vi "PickeringWriteConfig Asynchronous.vi"(8 "error in (no error)":errorcluster, 10 "Pickering Config":T1, 11 "Control Experiment in":refnum<class "Control Experiment.lvclass">) -> (0 "error out":errorcluster, 3 "Control Experiment out":refnum<class "Control Experiment.lvclass">)   [LabVIEW 2016, in "Control Experiment.lvclass"]
uses:
  Control Experiment.lvclass
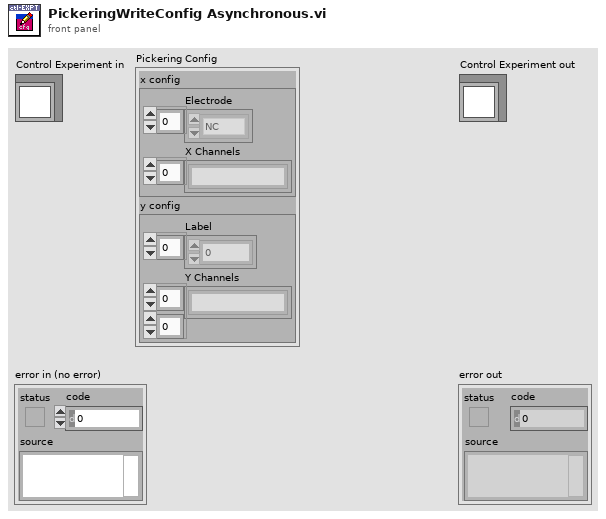
[diagram p1: front panel]
types:
  T1 = cluster{"x config":cluster{"Electrode":enum16{"NC", "26", "27", "28", "1", "2", "3", "4", "5", "6", "7", "8", "9", "10", "11", "12", "13", "14", "15", "16", "17", "18", "19", "20", "21", "22", "23", "24", "25"}[], "X Channels":string[]}, "y config":cluster{"Label":u16[], "Y Channels":string[][]}}
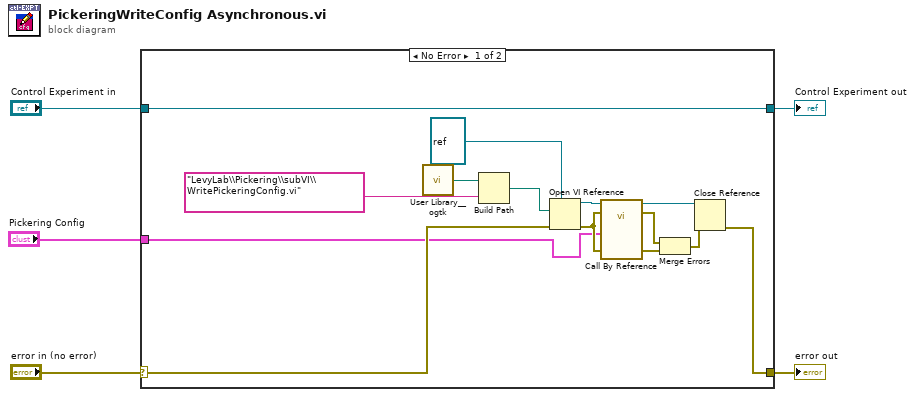
[diagram p0: block diagram]
diagram:
  n1 = case shown="No Error" "error in (no error)" {
    selector: "error in (no error)" -> [w9 w21]
    tunnel: [w8 w21] -> w4
    tunnel: [w19 w20] -> w2
    tunnel: "Control Experiment in" -> [w19 w20]
    tunnel: "Pickering Config" -> [w6 _]
    frame No Error {
      n2 = call <userlib>:"User Library__ogtk.vi"() -> ("User Library (+ Relative)"=w13:path)  [unwired: 1 in]
      n3 = Build Path(base path=w13, name or relative path="LevyLab\\Pickering\\subVI\\WritePickeringConfig.vi") -> (appended path=w10:path)
      n4 = Open VI Reference(type specifier VI Refnum (for type only)=refnum<vi> refnum, vi path=w10, error in (no error)=w9) -> (vi reference=w18:refnum<vi>, error out=w12:errorcluster)  [unwired: 3 in]
      n5 = call-by-ref "?"(reference=w18, error in=w12, 8:"error in (no error)"=w12, "Pickering Config"=w6) -> (reference out=w17:refnum<vi>, error out=w16:errorcluster, "Error Out"=w15:errorcluster)  [unwired: 9 in]
      n6 = Merge Errors(w16, w15) -> (w14:errorcluster)
      n7 = Close Reference(reference=w17, error in (no error)=w14) -> (error out=w8:errorcluster)
    }
    frame Error {
    }
  }
  "error out" <- w4
  "Control Experiment out" <- w2
